vi "Save Source in 2020.vi"() -> ()   [LabVIEW 2023]
panel:
  out "Number of Files converted":i32
  # "This VI saves the entire source in 2020. It should be ran before opening the VIPM build spec file. Once the build is made, the 2020 folder should be deleted."
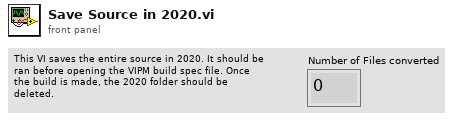
[diagram p1: front panel]
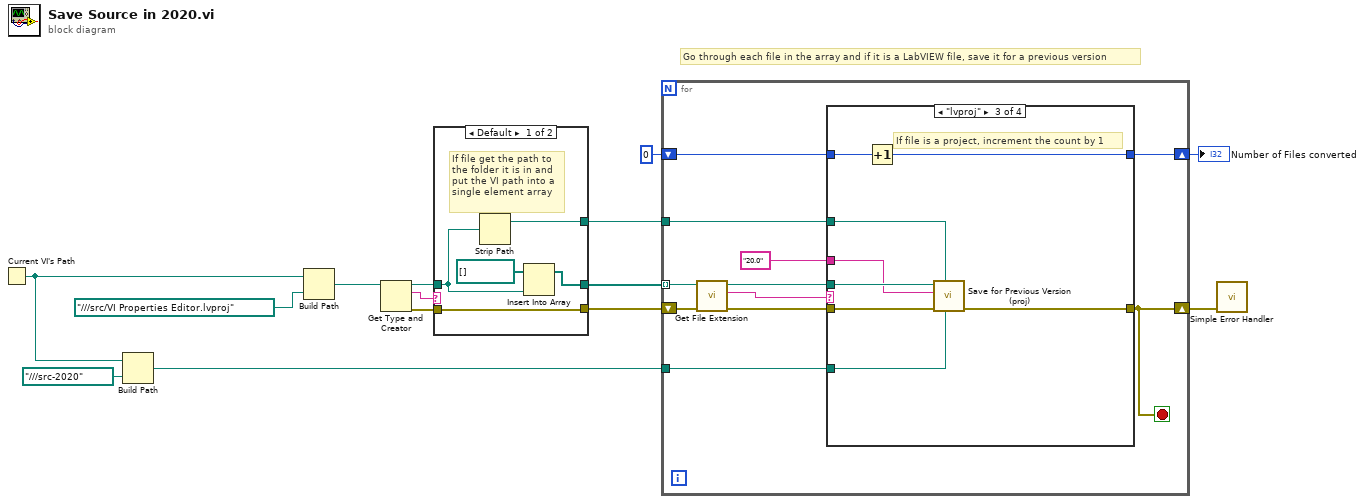
[diagram p0: block diagram]
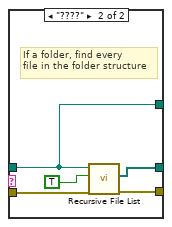
[diagram p2: hidden frame]
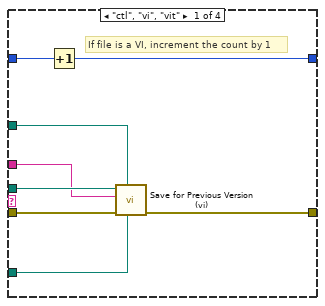
[diagram p3: hidden frame]
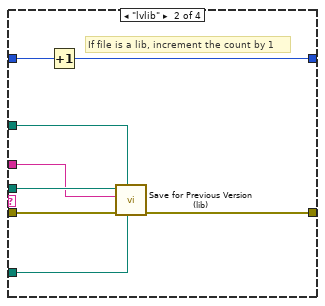
[diagram p4: hidden frame]
diagram:
  # "Go through each file in the array and if it is a LabVIEW file, save it for a previous version"
  n1 = Current VI's Path() -> (path=w12:path)
  n2 = Build Path(base path=w12, name or relative path=path "../../../src-2020") -> (appended path=w1:path)
  n3 = Build Path(base path=w12, name or relative path=path "../../../src/VI Properties Editor.lvproj") -> (appended path=w2:path)
  n4 = Get Type and Creator(7:w2) -> (0:w5:errorcluster, 2:w3:string, 3:w6:path)  [unwired: 1 in, 1 out]
  n5 = case shown="Default" w3 {
    tunnel: [w16 w24] -> w8
    tunnel: [w19 w23] -> w7
    tunnel: w6 -> [w18 w20]
    tunnel: w5 -> [w16 w21]
    tunnel: [w17 w20] -> w4
    frame Default {
      # "If file get the path to\nthe folder it is in and\nput the VI path into a\nsingle element array"
      n6 = Strip Path(path=w18) -> (stripped path=w17:path)  [unwired: 1 out]
      n7 = Insert Into Array(array=path[] [], new element=w18) -> (w19:path[])  [unwired: 1 in]
    }
    frame "????" {
      # "If a folder, find every\nfile in the folder structure"
      n8 = call <vilib>:"Recursive File List.vi"("error in (no error)"=w21, "Treat LLBs as Folders?"=TRUE, "Folder Path"=w20) -> ("error out"=w24:errorcluster, "All Files in Dir"=w23:path[])  [unwired: 4 in, 3 out]
    }
  }
  n9 = for {
    shift-right: [w29] -> w9
    shift-left: w8 -> [w35]
    shift-right: [w32] -> w10
    shift-left: 0 -> [w33]
    tunnel: w7 -> [w28] mode=indexing
    tunnel: w4 -> [w27]
    tunnel: w1 -> [w26]
    stop <- w29 stop-if-true
    n10 = call <vilib>:"Get File Extension.vi"("error in (no error)"=w35, "file"=w28) -> ("error out"=w34:errorcluster, "lowercase file extension"=w31:string, "dup file"=w30:path)  [unwired: 7 out]
    n11 = case shown="\"lvproj\"" w31 {
      tunnel: w33 -> [w43 w51 w59 w61]
      tunnel: [w42 w50 w58 w61] -> w32
      tunnel: w34 -> [w41 w49 w57 w60]
      tunnel: [w40 w48 w56 w60] -> w29
      tunnel: w30 -> [w39 w47 w55 _]
      tunnel: w27 -> [w38 w46 w54 _]
      tunnel: w26 -> [w37 w45 w53 _]
      tunnel: "20.0" -> [w36 w44 w52 _]
      frame "ctl", "vi", "vit" {
        # "If file is a VI, increment the count by 1"
        n12 = Increment(x=w43) -> (x+1=w42:i32)
        n13 = call "Save for Previous Version (vi).vi"("Destination Folder"=w37, "Folder to Convert"=w38, "error in (no error)"=w41, "Previous Version"=w36, "vi path"=w39) -> ("error out"=w40:errorcluster)  [unwired: 5 in, 1 out]
      }
      frame "lvlib" {
        # "If file is a lib, increment the count by 1"
        n14 = Increment(x=w51) -> (x+1=w50:i32)
        n15 = call "Save for Previous Version (lib).vi"("Destination Folder"=w45, "Folder to Convert"=w46, "error in (no error)"=w49, "Previous Version"=w44, "vi path"=w47) -> ("error out"=w48:errorcluster)  [unwired: 6 in]
      }
      frame "lvproj" {
        # "If file is a project, increment the count by 1"
        n16 = Increment(x=w59) -> (x+1=w58:i32)
        n17 = call "Save for Previous Version (proj).vi"("Destination Folder"=w53, "Folder to Convert"=w54, "error in (no error)"=w57, "Previous Version"=w52, "vi path"=w55) -> ("error out"=w56:errorcluster)  [unwired: 6 in]
      }
      frame "", Default {
        # "If file is not a VI or an LLB folder of VI's\ndo not increment the count"
      }
    }
  }
  "Number of Files converted" <- w10
  n18 = call <vilib>:"Simple Error Handler.vi"("error in (no error)"=w9) -> ()  [unwired: 4 in, 5 out]
